vi "readPress00.vi"() -> ()   [LabVIEW 2011]
panel:
  in  "y":i32=1000
  in  "VISA resource name":refnum<visa-resource-name>
  out "read buffer":string
  out "P (Torr)":dbl
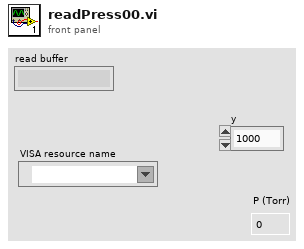
[diagram p1: front panel]
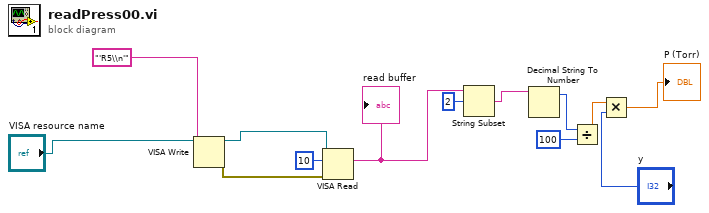
[diagram p0: block diagram]
diagram:
  n1 = VISA Write(VISA resource name="VISA resource name", write buffer="'R5\\n'") -> (VISA resource name out=w13:refnum<visa-resource-name>, error out=w9:errorcluster)  [unwired: 1 in, 1 out]
  n2 = VISA Read(VISA resource name=w13, byte count=u32 10, error in (no error)=w9) -> (read buffer=w12:string)  [unwired: 3 out]
  "read buffer" <- w12
  n3 = String Subset(string=w12, offset (0)=2) -> (substring=w11:string)  [unwired: 1 in]
  n4 = Decimal String To Number(string=w11) -> (offset past number=w4:i32)  [unwired: 2 in, 1 out]
  n5 = Divide(x=w4, y=100) -> (x/y=w2:dbl)
  n6 = Multiply(x=w2, y="y") -> (x*y=→"P (Torr)":dbl)
